vi "testUnflattenPressureFromXML.vi"() -> ()   [LabVIEW 2012, in "UnitsAndXML.lvlib"]
uses:
  <userlib>/Common/UnitsAndXML/UnitsAndXML.lvlib
  <userlib>/Common/UnitsAndXML/FlattenItemWithUnitToXML/FlattenPressureToXML/PressureUnit.ctl
  <userlib>/Common/UnitsAndXML/UnflattenItemWithUnitFromXML/UnflattenPressureFromXML/typeMethods/unflattenPressureFromXML_Array.vi
  <userlib>/Common/UnitsAndXML/UnflattenItemWithUnitFromXML/UnflattenPressureFromXML/typeMethods/unflattenPressureFromXML_Scalar.vi
panel:
  out "error out":errorcluster
  out "pressure":dbl[unit][](array[numeric])
  out "pressure":dbl[unit]
  in  "pressureUnitInXML":T1
  in  "xmlStringArray":string="<pressure>15</pressure>\r\n<pressure>30</pressure>\r\n<pressure>45</pressure>\r\n<pressure>60</pressure>"
  in  "xmlStringScalar":string="<pressure>15</pressure>"
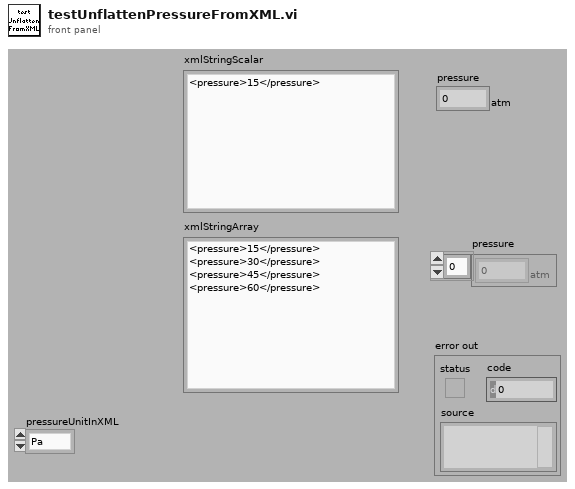
[diagram p1: front panel]
types:
  T1 = typedef "UnitsAndXML.lvlib/PressureUnit.ctl" = enum16{"Pa", "atm", "bar", "mbar", "m.Hg", "psi", "torr"}
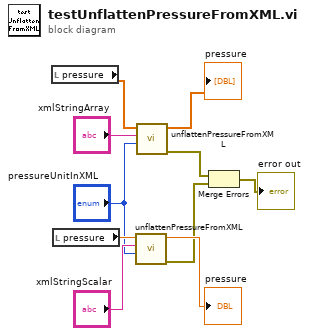
[diagram p0: block diagram]
diagram:
  n1 = local read "pressure"() -> (w3:dbl[unit][])
  n2 = local read "pressure"() -> (w9:dbl[unit])
  n3 = call-poly <userlib>:"unflattenPressureFromXML.vi"("pressureUnitInXML"="pressureUnitInXML", "xmlString"="xmlStringScalar", "pressureForType"=w9) -> ("error out"=w5:errorcluster, "pressure"=→"pressure":dbl[unit])  [unwired: 7 in]
  n4 = call-poly <userlib>:"unflattenPressureFromXML.vi"("pressureUnitInXML"="pressureUnitInXML", "xmlString"="xmlStringArray", "pressureForType"=w3) -> ("error out"=w6:errorcluster, "pressure"=→"pressure":dbl[unit][])  [unwired: 7 in]
  n5 = Merge Errors(w6, w5) -> (→"error out":errorcluster)
